vi "Do Write.vi"(8 "error in (no error)":errorcluster, 9 "Timeout ms":i32, 10 "Data":string, 11 "WebsocketStream in":refnum<class "WebsocketStream.lvclass">) -> (0 "error out":errorcluster, 1 "Remaining  Timeout":i32, 3 "WebsocketStream out":refnum<class "WebsocketStream.lvclass">)   [LabVIEW 2020, in "Stream-Websocket.lvlib" / "WebsocketStream.lvclass"]
uses:
  WebsocketStream.lvclass
  WebsocketStream.lvclass/WebsocketStream.ctl
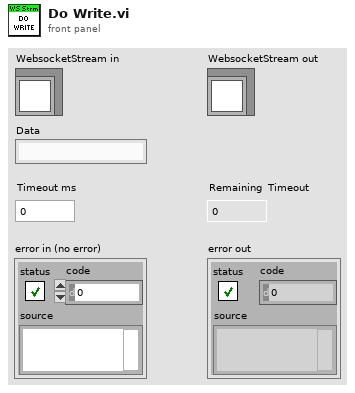
[diagram p1: front panel]
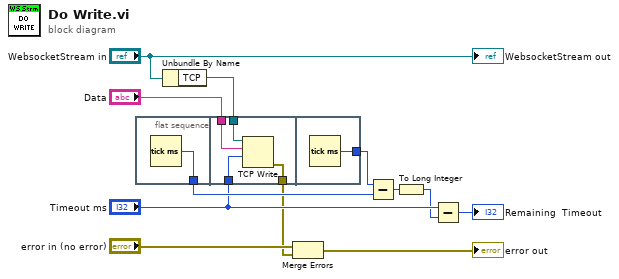
[diagram p0: block diagram]
diagram:
  n1 = flat-sequence {
    tunnel: [w13] -> w7
    tunnel: w10 -> [w17]
    tunnel: "Data" -> [w16]
    tunnel: "Timeout ms" -> [w15]
    tunnel: [w14] -> w1
    tunnel: [w18] -> w8
    frame #0 {
      n2 = Tick Count (ms)() -> (millisecond timer value=w13:u32)
    }
    frame #1 {
      n3 = TCP Write(connection ID=w17, data in=w16, 9:w15) -> (error out=w14:errorcluster)  [unwired: 1 in, 2 out]
    }
    frame #2 {
      n4 = Tick Count (ms)() -> (millisecond timer value=w18:u32)
    }
  }
  n5 = Unbundle By Name("WebsocketStream in") -> ("TCP"=w10:refnum<k5>)
  n6 = Merge Errors("error in (no error)", w1) -> (→"error out":errorcluster)
  n7 = Subtract(x=w8, y=w7) -> (x-y=w5:u32)
  n8 = To Long Integer(number=w5) -> (32bit integer=w4:i32)
  n9 = Subtract(x="Timeout ms", y=w4) -> (x-y=→"Remaining  Timeout":i32)
  "WebsocketStream out" <- "WebsocketStream in"
